vi "Parker Stepper Control.vi"(2 "Point #":i32, 4 "Parameters":dbl[](array[numeric]) format="%.3e", 5 "Instrument Address":refnum<visa-resource-name>) -> (0 "Stop":bool, 1 "Data Out":dbl[](array[numeric]) format="%.2f")   [LabVIEW 2019]
doc: "Moves the stepper moter an appropriate amount based on the point number, step size and final position.\nScott Hannahs, NHMFL, March 1999"
uses:
  Serial Support VISA.llb/Serial Actions.ctl
  Parker Stepper Global.vi
panel:
  out "Starting Position":dbl format="%.2f"
  # "Motor Number"
  # "Step Size"
  # "Final Position"
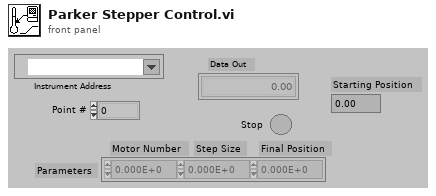
[diagram p1: front panel]
types:
  T1 = cluster{"Parameters[0]":dbl, "Parameters[1]":dbl, "Parameters[2]":dbl}
  T2 = typedef "Serial Actions.ctl" = enum16{"Init", "Break", "Clear Buffer", "Write", "Read", "N Bytes", "Lock", "Unlock", "Close"}
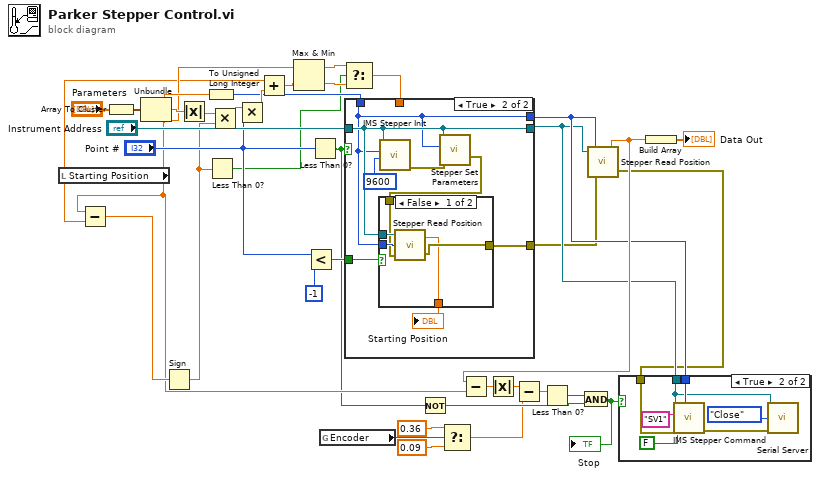
[diagram p0: block diagram]
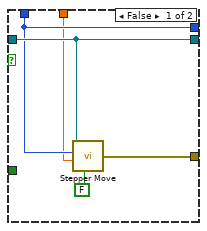
[diagram p3: hidden frame]
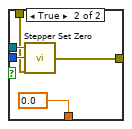
[diagram p4: hidden frame]
diagram:
  n1 = local read "Starting Position"() -> (w9:dbl)
  n2 = Array To Cluster(array="Parameters") -> (cluster=w37:T1)
  n3 = Unbundle(w37) -> ("Parameters[0]"=w34:dbl, "Parameters[1]"=w22:dbl, "Parameters[2]"=w15:dbl)
  n4 = Subtract(x=w15, y=w9) -> (x-y=w23:dbl)
  n5 = Sign(1:w23) -> (0:w14:dbl)
  n6 = Absolute Value(x=w22) -> (abs(x)=w20:dbl)
  n7 = To Unsigned Long Integer(number=w34) -> (unsigned 32bit integer=w28:u32)
  n8 = Less Than 0?(x=w14) -> (x < 0?=w13:bool)
  n9 = Multiply(x=w20, y=w14) -> (x*y=w21:dbl)
  n10 = Multiply(x=w21, y="Point #") -> (x*y=w36:dbl)
  n11 = Add(x=w9, y=w36) -> (x+y=w19:dbl)
  n12 = Max & Min(x=w15, y=w19) -> (max(x,y)=w17:dbl, min(x,y)=w16:dbl)
  n13 = Less?(x="Point #", y=-1) -> (x < y?=w25:bool)
  n14 = Less Than 0?(x="Point #") -> (x < 0?=w6:bool)
  n15 = global read "Parker Stepper Global.vi" "Encoder"() -> (w4:bool)
  n16 = Select(t=w17, s=w13, f=w16) -> (s? t:f=w18:dbl)
  n17 = case shown="True" w6 {
    tunnel: "Instrument Address" -> [w43 w45]
    tunnel: [w43 w45] -> w29
    tunnel: w28 -> [w42 w44]
    tunnel: [w42 w44] -> w30
    tunnel: [w41 w50] -> w10
    tunnel: w25 -> [_ w49]
    tunnel: w18 -> [w40 _]
    frame False {
      n18 = call "Stepper Move.vi"("Instrument Address"=w43, "Motor Number"=w42, "Distance"=w40, "Mode"=FALSE) -> ("error out"=w41:errorcluster)  [unwired: 1 in]
    }
    frame True {
      n19 = call "IMS Stepper Init.vi"("Baud Rate"=u32 9600, "Motor Number"=w44, "Instrument Address"=w45) -> ("error out"=w46:errorcluster)  [unwired: 2 in, 2 out]
      n20 = call "Stepper Set Parameters.vi"("error in (no error)"=w46, "Motor Number"=w44, "Instrument Address"=w45) -> ("error out"=w47:errorcluster)  [unwired: 3 in]
      n21 = case shown="False" w49 {
        tunnel: w44 -> [w56 w61]
        tunnel: w45 -> [w55 w60]
        tunnel: [w54 w59] -> w50
        tunnel: [w53 0.0] -> w48
        tunnel: w47 -> [w52 w57]
        frame False {
          n22 = call "Stepper Read Position.vi"("error in (no error)"=w52, "Motor Number"=w56, "Instrument Address"=w55) -> ("error out"=w54:errorcluster, "Response"=w53:dbl)
        }
        frame True {
          n23 = call "Stepper Set Zero.vi"("error in (no error)"=w57, "Motor Number"=w61, "Instrument Address"=w60) -> ("error out"=w59:errorcluster)
        }
      }
      "Starting Position" <- w48
    }
  }
  n24 = Not(x=w6) -> (.not. x?=w5:bool)
  n25 = Select(t=0.36 ("y"), s=w4, f=0.09 ("y")) -> (s? t:f=w1:dbl)
  n26 = call "Stepper Read Position.vi"("error in (no error)"=w10, "Motor Number"=w30, "Instrument Address"=w29) -> ("error out"=w24:errorcluster, "Response"=w32:dbl)
  n27 = Subtract(x=w32, y=w15) -> (x-y=w31:dbl)
  n28 = Absolute Value(x=w31) -> (abs(x)=w12:dbl)
  n29 = Subtract(x=w12, y=w1) -> (x-y=w11:dbl)
  n30 = Less Than 0?(x=w11) -> (x < 0?=w7:bool)
  n31 = And(x=w7, y=w5) -> (x .and. y?=w8:bool)
  "Stop" <- w8
  n32 = case shown="True" w8 {
    tunnel: w30 -> [_ w65]
    tunnel: w29 -> [_ w62]
    tunnel: w24 -> [_ w67]
    frame False {
    }
    frame True {
      n33 = call "IMS Stepper Command.vi"("Motor Number"=w65, "error in (no error)"=w67, "Mode"=FALSE, "Command"="SV1", "Instrument Address"=w62) -> ("error out"=w66:errorcluster)  [unwired: 1 in, 3 out]
      n34 = call "Serial Server.vi"("VISA Resource Name"=w62, "Action"=Serial_Actions."Close", "error in (no error)"=w66) -> ()  [unwired: 8 in, 5 out]
    }
  }
  n35 = Build Array(w32) -> (→"Data Out":dbl[])
